vi "ILABs_CaseHandler.vi"(2 "error In":errorcluster, 3 "appReference":refnum<vi>, 4 "data":string, 5 "action":string) -> (0 "errorOut":string, 1 "response":string)   [LabVIEW 2009]
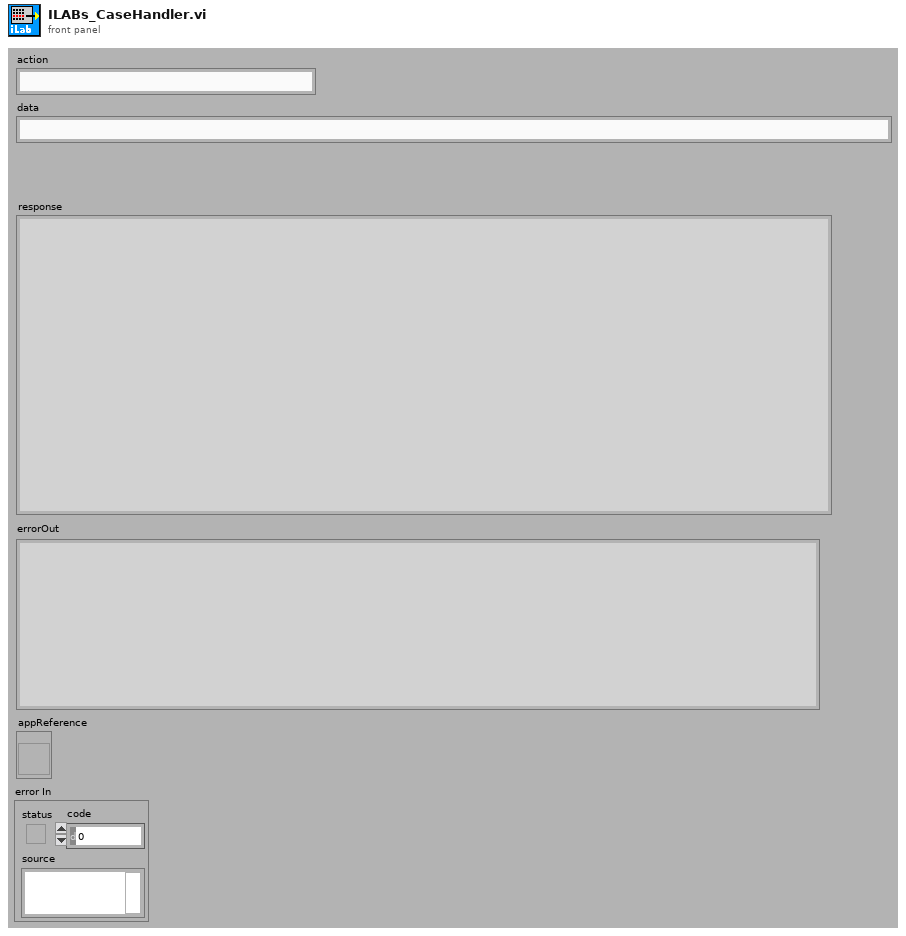
[diagram p1: front panel]
types:
  T1 = enum32{"Bad", "Idle", "Run top level", "Running"}
  T2 = typedef "LVRemotePanelConnectionsTypeDef.ctl" = cluster{"VI Name":string, "Remote":string, "UserName":string, "Port":i32, "Status":enum32{"Viewing", "Waiting For Control", "Controlling"}, "Create Time":timestamp, "Status Time":timestamp, "Control End Time":timestamp}[]
  T3 = cluster{"VI Name":string, "Remote":string, "UserName":string, "Port":i32, "Status":enum32{"Viewing", "Waiting For Control", "Controlling"}, "Create Time":timestamp, "Status Time":timestamp, "Control End Time":timestamp}
  T4 = cluster{"Name":string, "Path":path, "Type String":string, "Display Name":string, "Type":string}
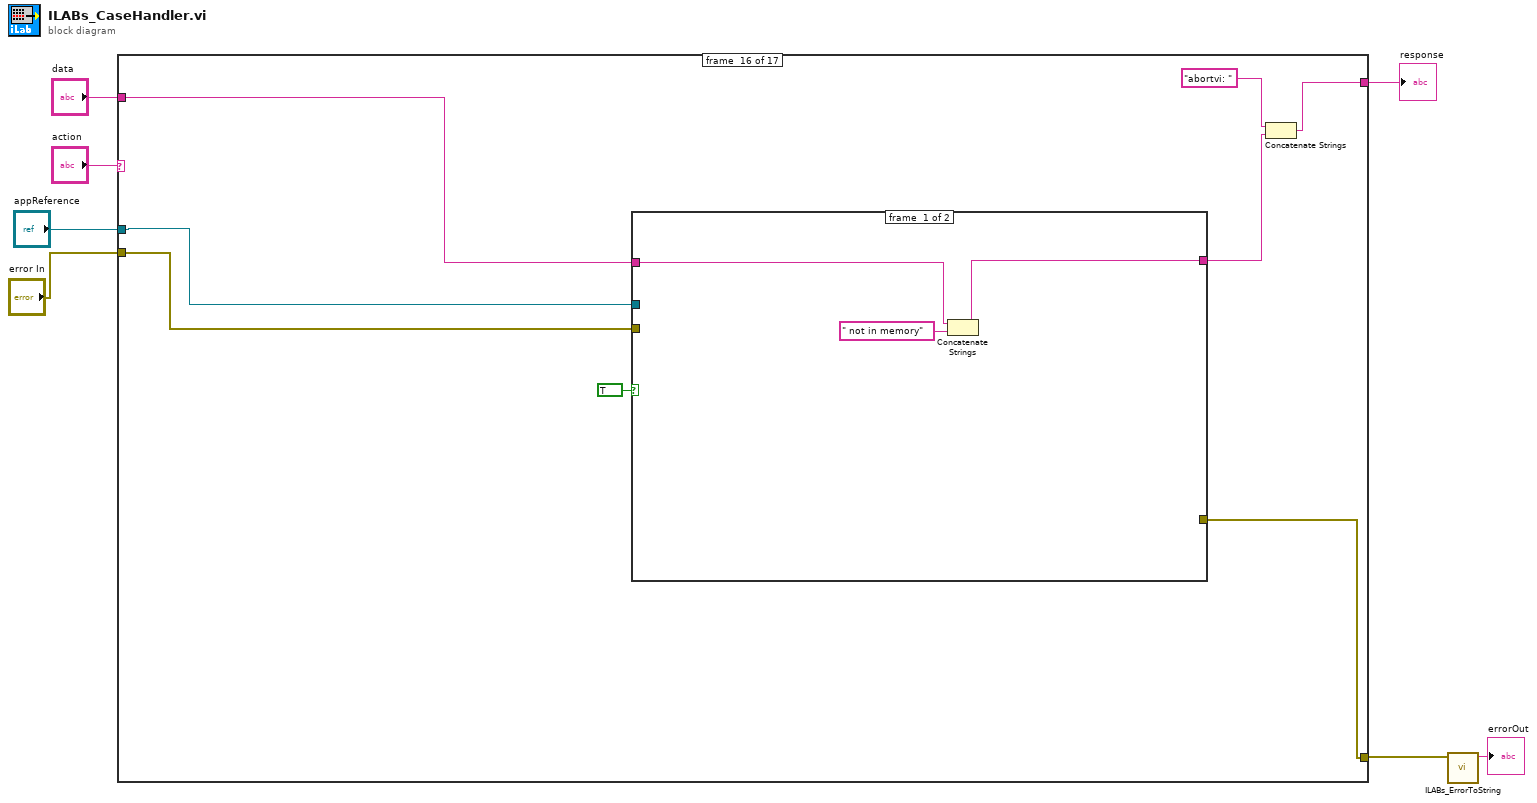
[diagram p0: block diagram]
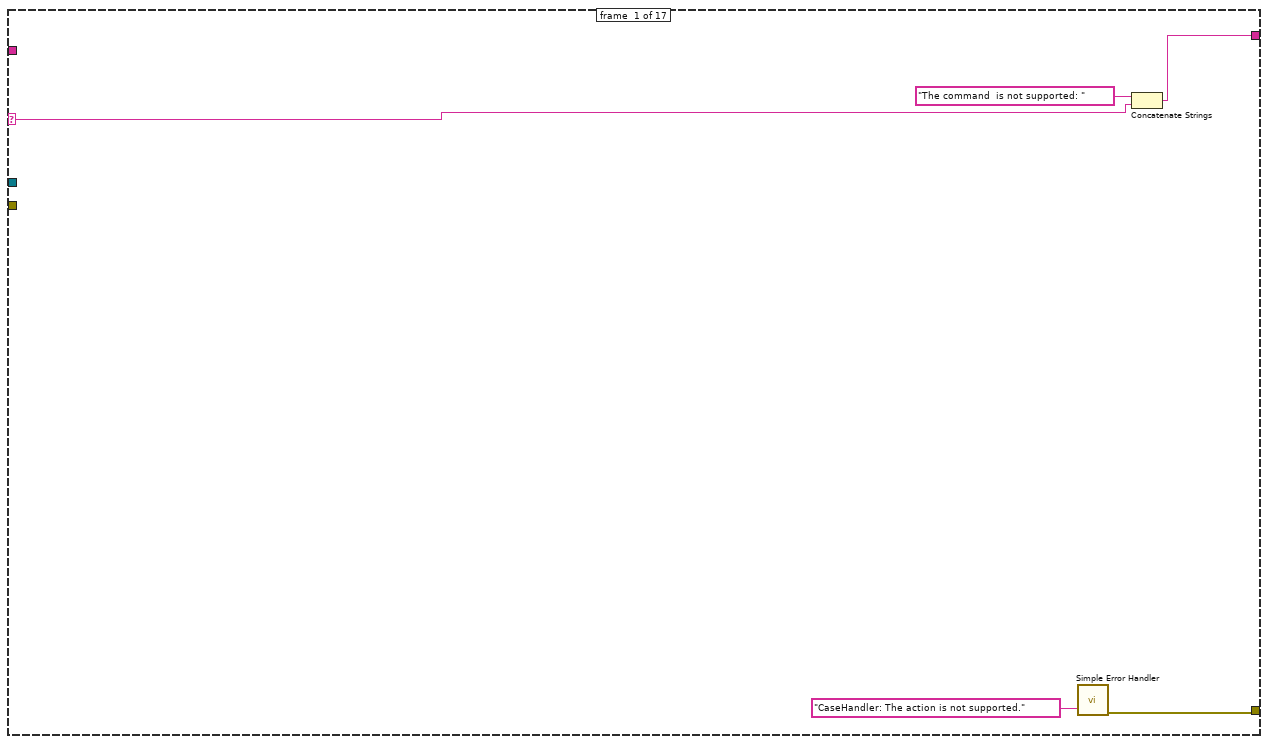
[diagram p2: hidden frame]
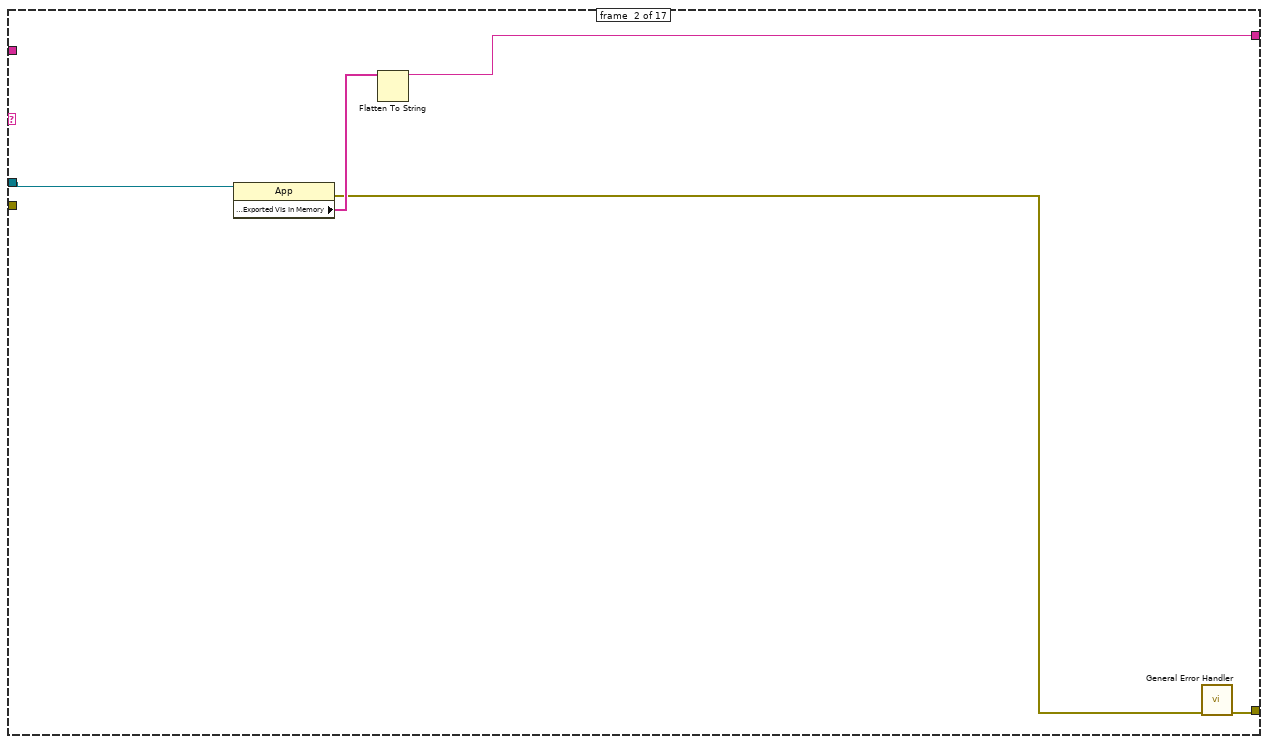
[diagram p3: hidden frame]
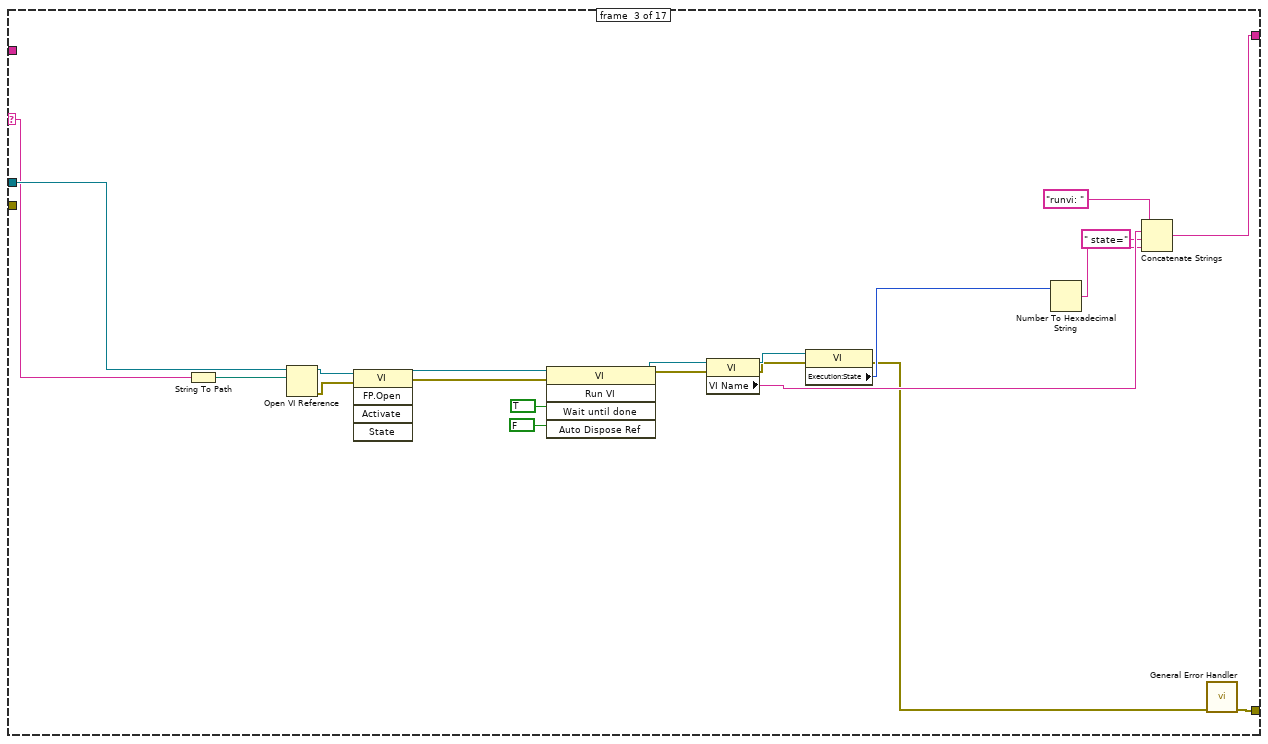
[diagram p4: hidden frame]
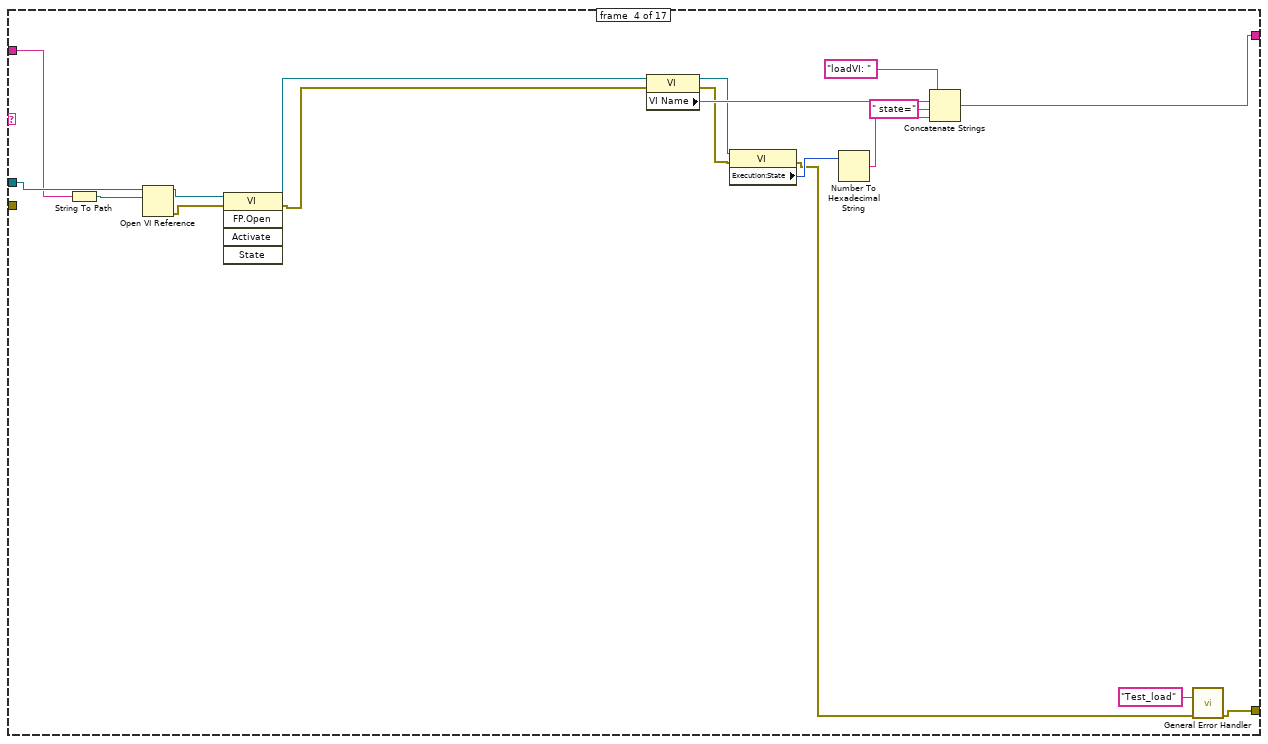
[diagram p5: hidden frame]
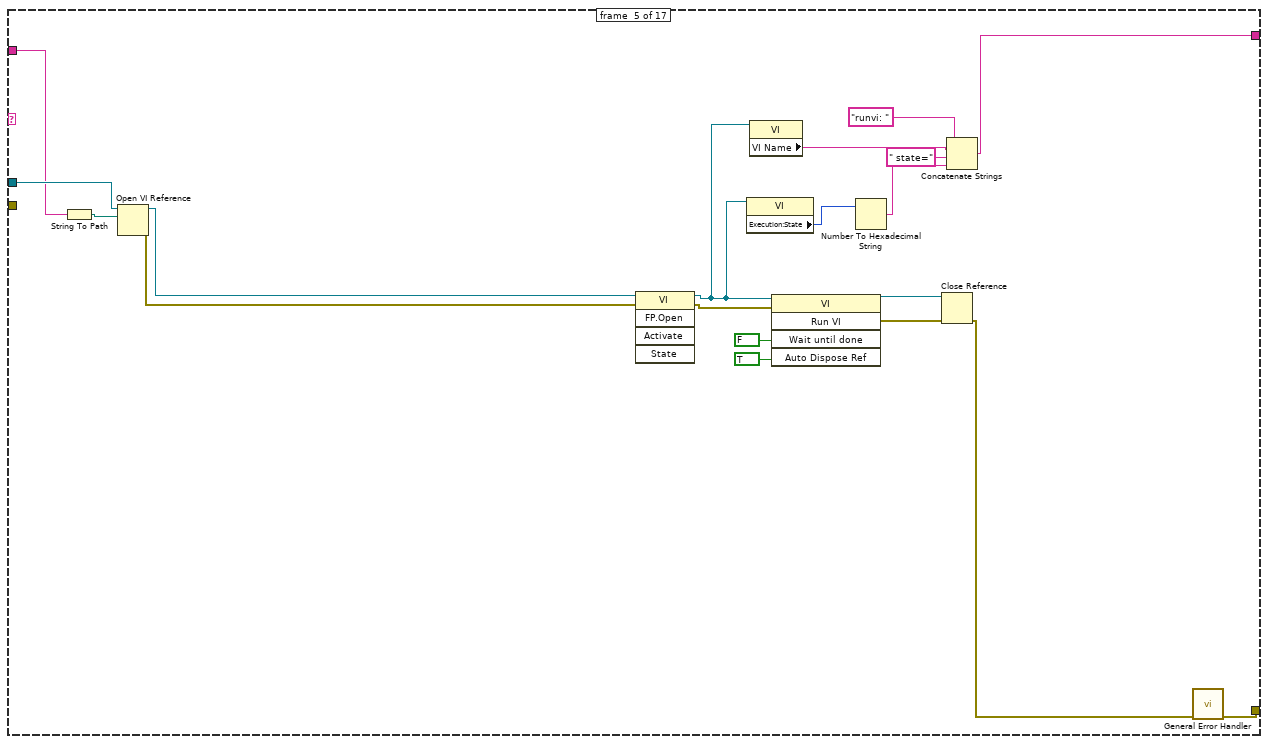
[diagram p6: hidden frame]
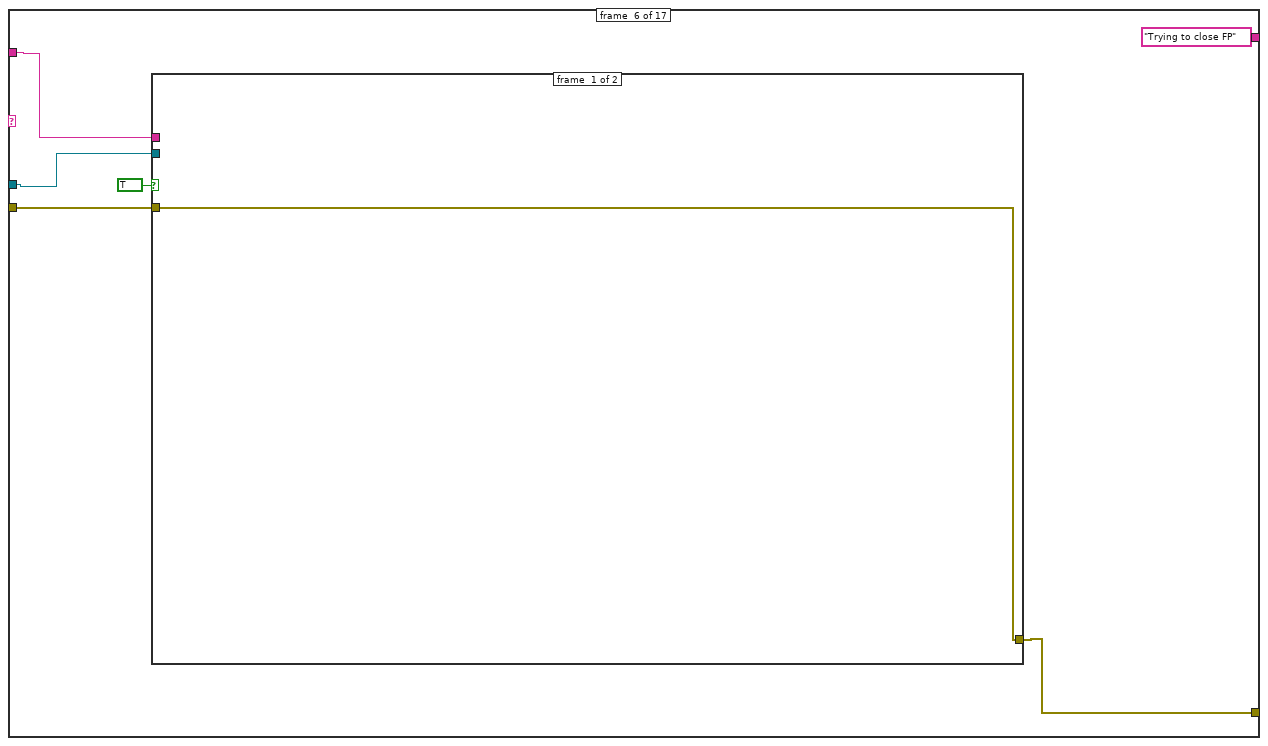
[diagram p7: hidden frame]
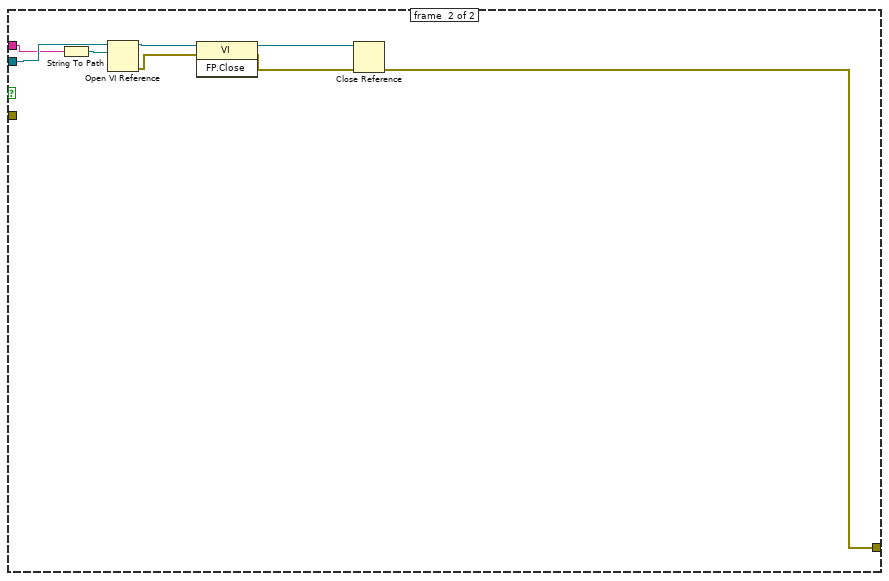
[diagram p8: hidden frame]
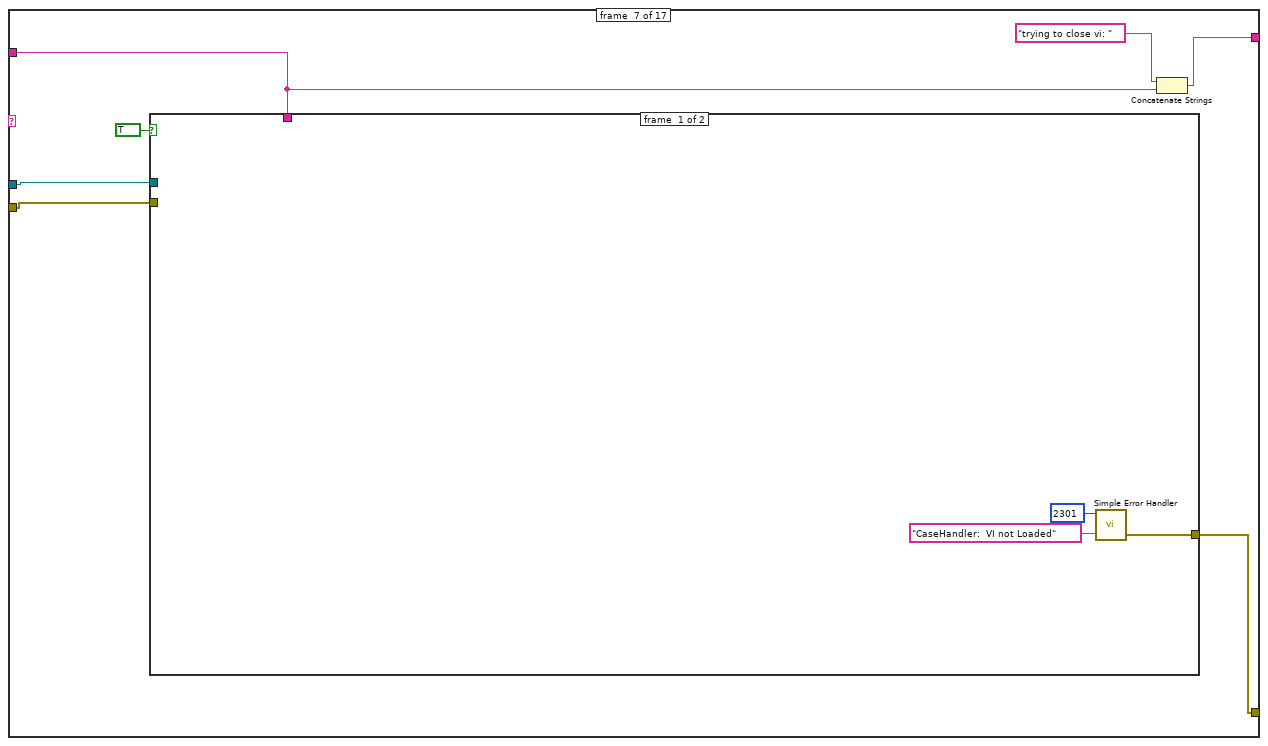
[diagram p9: hidden frame]
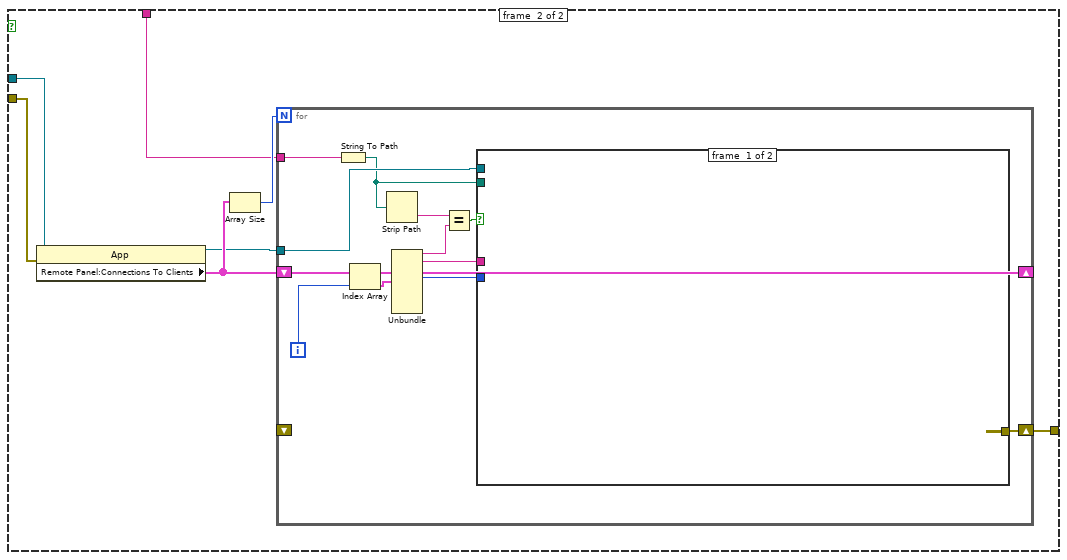
[diagram p10: hidden frame]
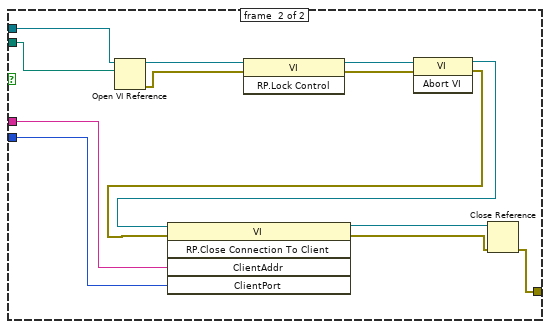
[diagram p11: hidden frame]
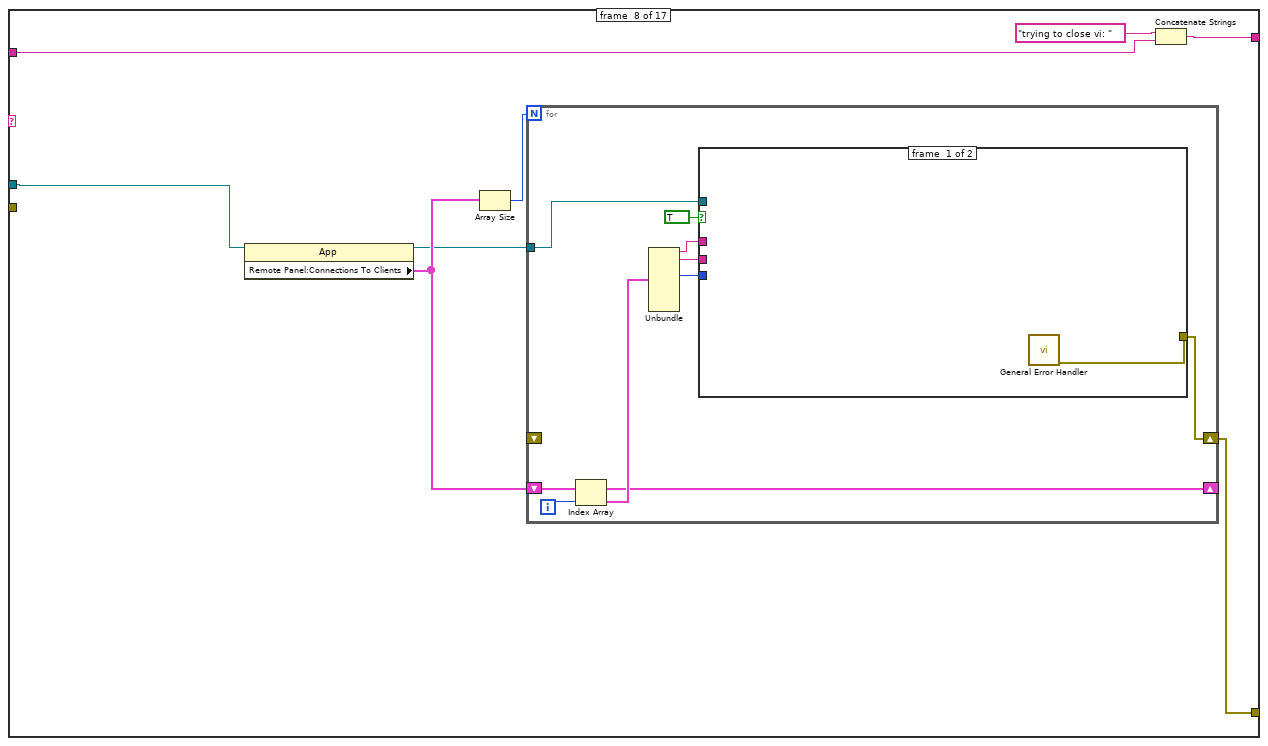
[diagram p12: hidden frame]
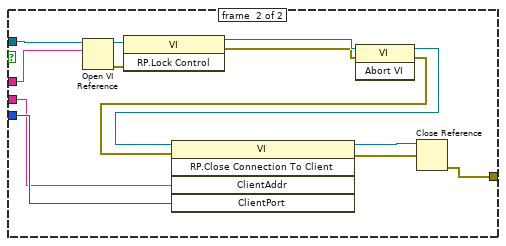
[diagram p13: hidden frame]
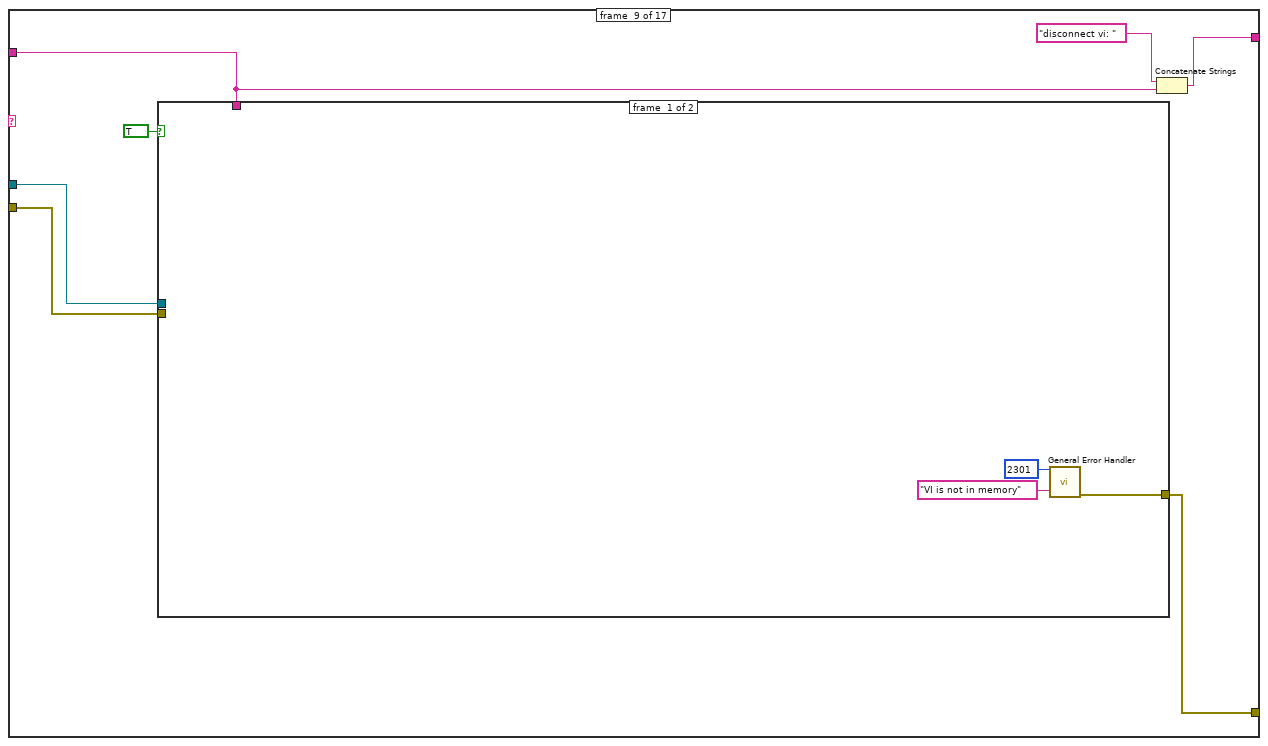
[diagram p14: hidden frame]
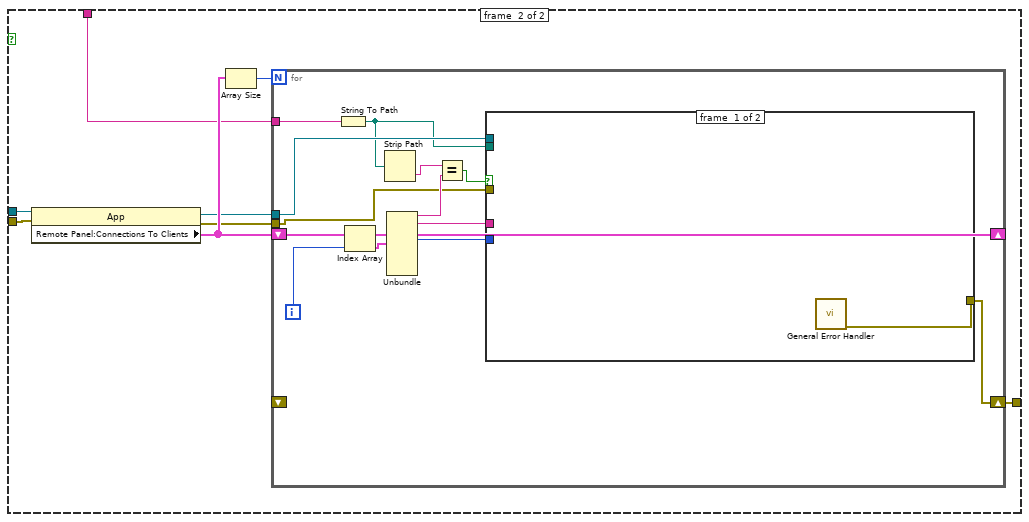
[diagram p15: hidden frame]
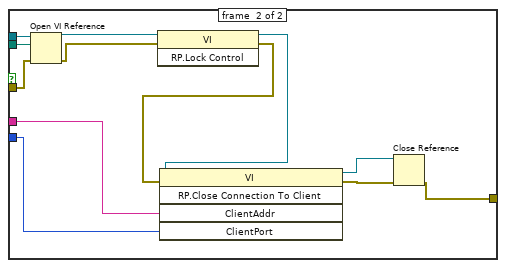
[diagram p16: hidden frame]
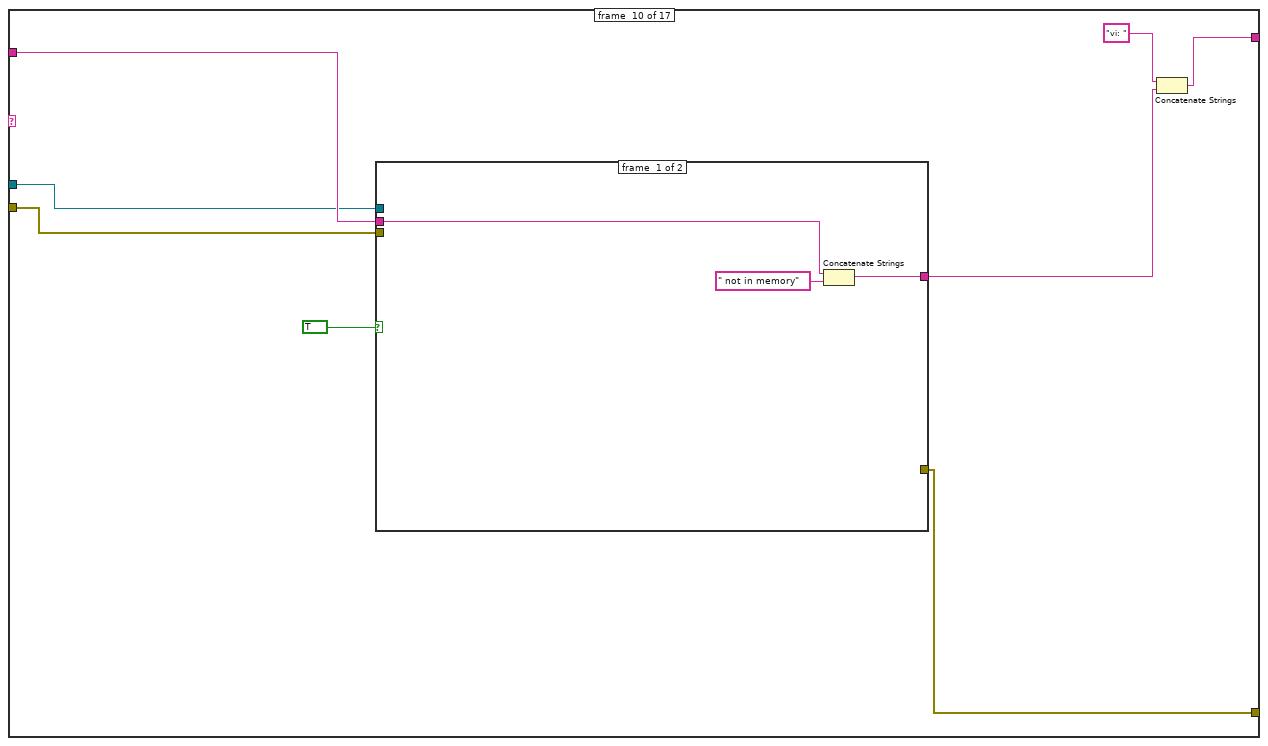
[diagram p17: hidden frame]
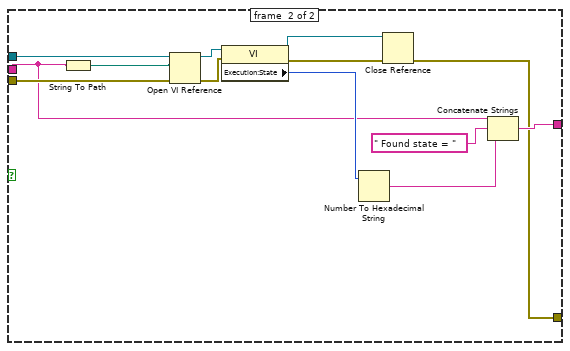
[diagram p18: hidden frame]
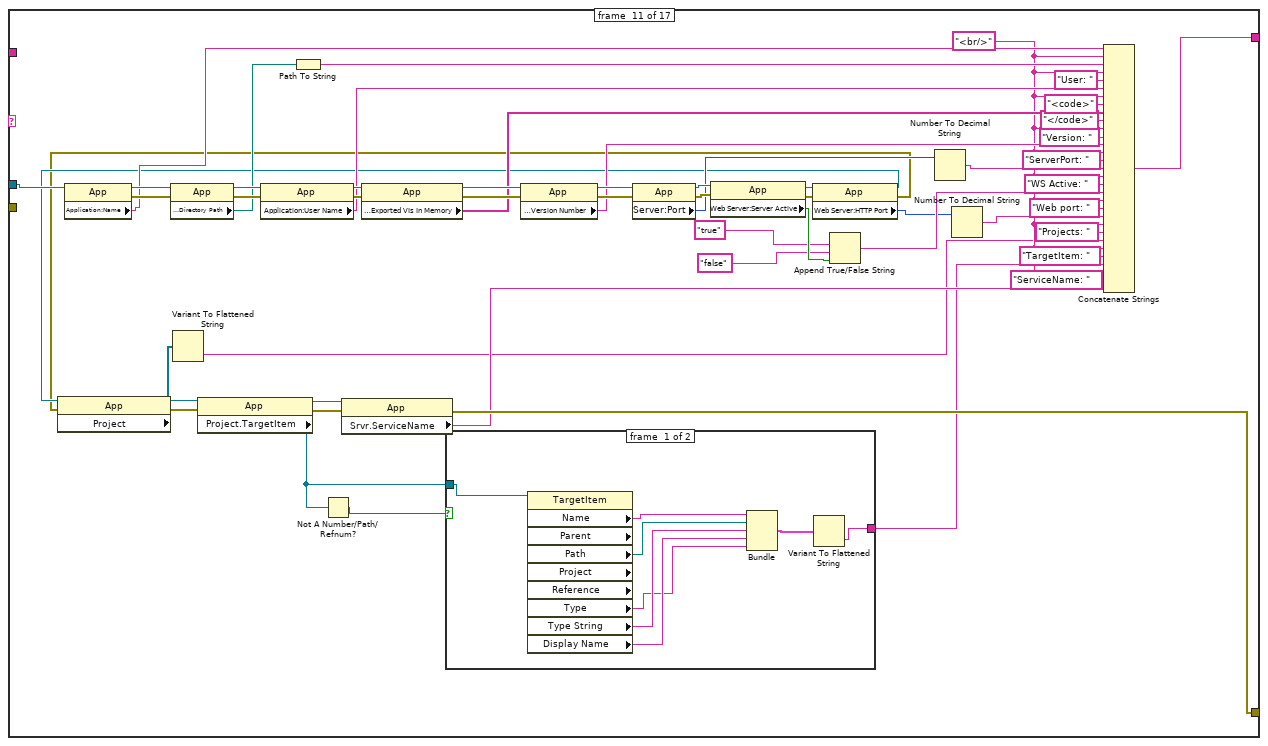
[diagram p19: hidden frame]
diagram:
  n1 = case shown="\"appstatus\"" "action" {
    selector: "action" -> [w11 _ w18 _ _ _ _ _ _ _ _ _ _ _ _ _ _]
    tunnel: "data" -> [_ _ _ w39 w57 w81 w94 w137 w167 w212 _ w295 w317 w327 w342 w370 w394]
    tunnel: [w10 w17 w30 w50 w66 "Trying to close FP" ("data") w96 w136 w169 w215 w249 w306 w326 w338 w346 w374 w394] -> w6
    tunnel: [w8 w14 w28 w49 w63 w79 w95 w135 w168 w211 w242 w297 w318 w329 w343 w371 _] -> w4
    tunnel: "appReference" -> [_ w13 w27 w48 w62 w80 w93 w134 w166 w210 w285 w294 w311 w330 w341 w369 _]
    tunnel: "error In" -> [_ _ _ _ _ w76 w92 _ w164 w209 _ w299 w312 _ w340 w368 _]
    frame #0 {
      (unwired) "The" ("message")
      n2 = call <vilib>:"Simple Error Handler.vi"("error source (\" \")"="CaseHandler: The action is not supported." ("error source (\" \")")) -> ("error out"=w8:errorcluster)  [unwired: 2 in, 6 out]
      n3 = Concatenate Strings("The command  is not supported: " ("string"), w11) -> (w10:string)
    }
    frame #1 {
      n4 = property class="App"(reference=w13) -> (error out=w15:errorcluster, "Application:Exported VIs In Memory"=w16:string[])  [unwired: 1 in, 1 out]
      n5 = Flatten To String(anything=w16) -> (data string=w17:string)  [unwired: 1 in, 4 out]
      n6 = call <vilib>:"General Error Handler.vi"("error in (no error)"=w15) -> ("error out"=w14:errorcluster)  [unwired: 1 in, 13 out]
    }
    frame #2 {
      n7 = String To Path(string=w18) -> (path=w19:path)
      n8 = Open VI Reference(application reference (local)=w27, vi path=w19) -> (vi reference=w37:refnum<vi>, error out=w36:errorcluster)  [unwired: 1 in, 3 out]
      n9 = invoke class="VI" method="FP.Open"(reference=w37, error in=w36) -> (reference out=w26:refnum<vi>, error out=w25:errorcluster)  [unwired: 3 in, 3 out]
      n10 = invoke class="VI" method="Run VI"(reference=w26, error in=w25, "Wait until done"=FALSE, "Auto Dispose Ref"=TRUE) -> (reference out=w24:refnum<vi>, error out=w23:errorcluster)  [unwired: 1 in, 3 out]
      n11 = property class="VI"(reference=w24, error in=w23) -> (reference out=w22:refnum<vi>, error out=w21:errorcluster, "VI Name"=w35:string)
      n12 = property class="VI"(reference=w22, error in=w21) -> (error out=w20:errorcluster, "Execution:State"=w33:T1)  [unwired: 1 out]
      n13 = Number To Hexadecimal String(2:w33) -> (0:w32:string)  [unwired: 1 out]
      n14 = Concatenate Strings("runvi: " ("string"), w35, " state=" ("string"), w32) -> (w30:string)
      n15 = call <vilib>:"General Error Handler.vi"("error in (no error)"=w20) -> ("error out"=w28:errorcluster)  [unwired: 1 in, 13 out]
    }
    frame #3 {
      n16 = String To Path(string=w39) -> (path=w40:path)
      n17 = Open VI Reference(application reference (local)=w48, vi path=w40) -> (vi reference=w44:refnum<vi>, error out=w43:errorcluster)  [unwired: 1 in, 3 out]
      n18 = invoke class="VI" method="FP.Open"(reference=w44, error in=w43) -> (reference out=w42:refnum<vi>, error out=w41:errorcluster)  [unwired: 3 in, 3 out]
      n19 = property class="VI"(reference=w42, error in=w41) -> (reference out=w46:refnum<vi>, error out=w47:errorcluster, "VI Name"=w55:string)
      n20 = property class="VI"(reference=w46, error in=w47) -> (error out=w45:errorcluster, "Execution:State"=w53:T1)  [unwired: 1 out]
      n21 = Number To Hexadecimal String(2:w53) -> (0:w52:string)  [unwired: 1 out]
      n22 = Concatenate Strings("loadVI: " ("string"), w55, " state=" ("string"), w52) -> (w50:string)
      n23 = call <vilib>:"General Error Handler.vi"("[error source] (\" \")"="Test_load" ("[error source] (\" \")"), "error in (no error)"=w45) -> ("error out"=w49:errorcluster)  [unwired: 1 in, 12 out]
    }
    frame #4 {
      w64 = TRUE items=["OFF", "ON", "OFF", "ON"] ("Auto Dispose Ref")
      n24 = String To Path(string=w57) -> (path=w58:path)
      n25 = Open VI Reference(application reference (local)=w62, vi path=w58) -> (vi reference=w74:refnum<vi>, error out=w72:errorcluster)  [unwired: 1 in, 3 out]
      n26 = invoke class="VI" method="FP.Open"(reference=w74, error in=w72) -> (reference out=w71:refnum<vi>, error out=w73:errorcluster)  [unwired: 3 in, 3 out]
      n27 = property class="VI"(reference=w71) -> ("Execution:State"=w68:T1)  [unwired: 1 in, 2 out]
      n28 = property class="VI"(reference=w71) -> ("VI Name"=w70:string)  [unwired: 1 in, 2 out]
      n29 = invoke class="VI" method="Run VI"(reference=w71, error in=w73, "Wait until done"=FALSE, "Auto Dispose Ref"=w64) -> (reference out=w59:refnum<vi>, error out=w60:errorcluster)  [unwired: 1 in, 3 out]
      n30 = Number To Hexadecimal String(2:w68) -> (0:w67:string)  [unwired: 1 out]
      n31 = Close Reference(reference=w59, error in (no error)=w60) -> (error out=w61:errorcluster)
      n32 = Concatenate Strings("runvi: " ("string"), w70, " state=" ("string"), w67) -> (w66:string)
      n33 = call <vilib>:"General Error Handler.vi"("error in (no error)"=w61) -> ("error out"=w63:errorcluster)  [unwired: 1 in, 13 out]
    }
    frame #5 {
      n34 = case shown="True" TRUE {
        tunnel: w81 -> [_ w83]
        tunnel: w80 -> [_ w90]
        tunnel: [w82 w85] -> w79
        tunnel: w76 -> [w82 _]
        frame #0 {
        }
        frame #1 {
          n35 = String To Path(string=w83) -> (path=w84:path)
          n36 = Open VI Reference(application reference (local)=w90, vi path=w84) -> (vi reference=w89:refnum<vi>, error out=w88:errorcluster)  [unwired: 1 in, 3 out]
          n37 = invoke class="VI" method="FP.Close"(reference=w89, error in=w88) -> (reference out=w87:refnum<vi>, error out=w86:errorcluster)  [unwired: 1 in, 1 out]
          n38 = Close Reference(reference=w87, error in (no error)=w86) -> (error out=w85:errorcluster)
        }
      }
    }
    frame #6 {
      n39 = case shown="True" TRUE {
        tunnel: [w100 w105] -> w95
        tunnel: w94 -> [_ w104]
        tunnel: w92 -> [_ w102]
        tunnel: w93 -> [_ w103]
        frame #0 {
          n40 = call <vilib>:"Simple Error Handler.vi"("error code (no error:0)"=2301, "error source (\" \")"="CaseHandler:  VI not Loaded" ("error source (\" \")")) -> ("error out"=w100:errorcluster)  [unwired: 2 in, 5 out]
        }
        frame #1 {
          n41 = property class="App"(reference=w103, error in=w102) -> (reference out=w101:refnum<vi>, "Remote Panel:Connections To Clients"=w106:T2)  [unwired: 1 out]
          n42 = Array Size(array=w106) -> (size(s)=w107:i32)
          n43 = for {
            N: w107 -> [_]
            shift-right: [w112] -> _
            shift-left: w106 -> [w112]
            tunnel: w104 -> [w109]
            shift-right: [w114] -> w105
            shift-left: _ -> [_]
            tunnel: w101 -> [w111]
            i -> [w119]
            n44 = String To Path(string=w109) -> (path=w108:path)
            n45 = Index Array(array=w112, index=w119) -> (element=w118:T3)
            n46 = Strip Path(path=w108) -> (name=w110:string)  [unwired: 1 out]
            n47 = Unbundle(w118) -> ("VI Name"=w113:string, "Remote"=w115:string, "Port"=w116:i32)  [unwired: 5 out]
            n48 = Equal?(x=w110, y=w113) -> (x = y?=w117:bool)
            n49 = case shown="True" w117 {
              tunnel: w116 -> [_ w132]
              tunnel: w115 -> [_ w131]
              tunnel: [_ w130] -> w114
              tunnel: w111 -> [_ w121]
              tunnel: w108 -> [_ w120]
              frame #0 {
              }
              frame #1 {
                n50 = Open VI Reference(application reference (local)=w121, vi path=w120) -> (vi reference=w129:refnum<vi>, error out=w128:errorcluster)  [unwired: 1 in, 3 out]
                n51 = invoke class="VI" method="RP.Lock Control"(reference=w129, error in=w128) -> (reference out=w127:refnum<vi>, error out=w126:errorcluster)  [unwired: 1 in, 1 out]
                n52 = invoke class="VI" method="Abort VI"(reference=w127, error in=w126) -> (reference out=w123:refnum<vi>, error out=w125:errorcluster)  [unwired: 1 in, 1 out]
                n53 = invoke class="VI" method="RP.Close Connection To Client"(reference=w123, error in=w125, "ClientAddr"=w131, "ClientPort"=w132) -> (reference out=w122:refnum<vi>, error out=w124:errorcluster)  [unwired: 1 in, 3 out]
                n54 = Close Reference(reference=w122, error in (no error)=w124) -> (error out=w130:errorcluster)
              }
            }
          }
        }
      }
      n55 = Concatenate Strings("trying to close vi: " ("data"), w94) -> (w96:string)
    }
    frame #7 {
      n56 = property class="App"(reference=w134) -> (reference out=w133:refnum<vi>, "Remote Panel:Connections To Clients"=w139:T2)  [unwired: 1 in, 1 out]
      n57 = Array Size(array=w139) -> (size(s)=w140:i32)
      n58 = for {
        N: w140 -> [_]
        shift-right: [w143] -> _
        shift-left: w139 -> [w143]
        shift-right: [w145] -> w135
        shift-left: _ -> [_]
        tunnel: w133 -> [w142]
        i -> [w149]
        n59 = Index Array(array=w143, index=w149) -> (element=w148:T3)
        n60 = Unbundle(w148) -> ("VI Name"=w144:string, "Remote"=w146:string, "Port"=w147:i32)  [unwired: 5 out]
        n61 = case shown="True" TRUE {
          tunnel: w147 -> [_ w163]
          tunnel: w146 -> [_ w162]
          tunnel: [w150 w161] -> w145
          tunnel: w144 -> [_ w160]
          tunnel: w142 -> [_ w151]
          frame #0 {
            n62 = call <vilib>:"General Error Handler.vi"() -> ("error out"=w150:errorcluster)  [unwired: 2 in, 13 out]
          }
          frame #1 {
            n63 = Open VI Reference(application reference (local)=w151, vi path=w160) -> (vi reference=w155:refnum<vi>, error out=w154:errorcluster)  [unwired: 1 in, 3 out]
            n64 = invoke class="VI" method="RP.Lock Control"(reference=w155, error in=w154) -> (reference out=w153:refnum<vi>, error out=w152:errorcluster)  [unwired: 1 in, 1 out]
            n65 = invoke class="VI" method="Abort VI"(reference=w153, error in=w152) -> (reference out=w156:refnum<vi>, error out=w157:errorcluster)  [unwired: 1 in, 1 out]
            n66 = invoke class="VI" method="RP.Close Connection To Client"(reference=w156, error in=w157, "ClientAddr"=w162, "ClientPort"=w163) -> (reference out=w159:refnum<vi>, error out=w158:errorcluster)  [unwired: 1 in, 3 out]
            n67 = Close Reference(reference=w159, error in (no error)=w158) -> (error out=w161:errorcluster)
          }
        }
      }
      n68 = Concatenate Strings("trying to close vi: " ("data"), w137) -> (w136:string)
    }
    frame #8 {
      n69 = case shown="True" TRUE {
        tunnel: [w173 w179] -> w168
        tunnel: w167 -> [_ w178]
        tunnel: w166 -> [_ w177]
        tunnel: w164 -> [_ w175]
        frame #0 {
          n70 = call <vilib>:"General Error Handler.vi"("[error code] (0)"=2301, "[error source] (\" \")"="VI is not in memory" ("[error source] (\" \")")) -> ("error out"=w173:errorcluster)  [unwired: 2 in, 11 out]
        }
        frame #1 {
          n71 = property class="App"(reference=w177, error in=w175) -> (reference out=w176:refnum<vi>, error out=w174:errorcluster, "Remote Panel:Connections To Clients"=w180:T2)
          n72 = Array Size(array=w180) -> (size(s)=w181:i32)
          n73 = for {
            N: w181 -> [_]
            shift-right: [w187] -> _
            shift-left: w180 -> [w187]
            tunnel: w178 -> [w183]
            shift-right: [w189] -> w179
            shift-left: _ -> [_]
            tunnel: w176 -> [w186]
            tunnel: w174 -> [w185]
            i -> [w194]
            n74 = String To Path(string=w183) -> (path=w182:path)
            n75 = Index Array(array=w187, index=w194) -> (element=w193:T3)
            n76 = Strip Path(path=w182) -> (name=w184:string)  [unwired: 1 out]
            n77 = Unbundle(w193) -> ("VI Name"=w188:string, "Remote"=w190:string, "Port"=w191:i32)  [unwired: 5 out]
            n78 = Equal?(x=w184, y=w188) -> (x = y?=w192:bool)
            n79 = case shown="True" w192 {
              tunnel: w191 -> [_ w207]
              tunnel: w190 -> [_ w206]
              tunnel: [w195 w198] -> w189
              tunnel: w186 -> [_ w201]
              tunnel: w185 -> [_ w197]
              tunnel: w182 -> [_ w196]
              frame #0 {
                n80 = call <vilib>:"General Error Handler.vi"() -> ("error out"=w195:errorcluster)  [unwired: 2 in, 13 out]
              }
              frame #1 {
                n81 = Open VI Reference(application reference (local)=w201, vi path=w196, error in (no error)=w197) -> (vi reference=w205:refnum<vi>, error out=w202:errorcluster)  [unwired: 3 out]
                n82 = invoke class="VI" method="RP.Lock Control"(reference=w205, error in=w202) -> (reference out=w204:refnum<vi>, error out=w203:errorcluster)  [unwired: 1 in, 1 out]
                n83 = invoke class="VI" method="RP.Close Connection To Client"(reference=w204, error in=w203, "ClientAddr"=w206, "ClientPort"=w207) -> (reference out=w199:refnum<vi>, error out=w200:errorcluster)  [unwired: 1 in, 3 out]
                n84 = Close Reference(reference=w199, error in (no error)=w200) -> (error out=w198:errorcluster)
              }
            }
          }
        }
      }
      n85 = Concatenate Strings("disconnect vi: " ("data"), w167) -> (w169:string)
    }
    frame #9 {
      n86 = case shown="True" TRUE {
        tunnel: w212 -> [w218 w220]
        tunnel: [_ w222] -> w211
        tunnel: [w217 w227] -> w213
        tunnel: w210 -> [_ w225]
        tunnel: w209 -> [_ w221]
        frame #0 {
          n87 = Concatenate Strings(w218, " not in memory" ("string")) -> (w217:string)
        }
        frame #1 {
          n88 = String To Path(string=w220) -> (path=w219:path)
          n89 = Open VI Reference(application reference (local)=w225, vi path=w219, error in (no error)=w221) -> (vi reference=w231:refnum<vi>, error out=w230:errorcluster)  [unwired: 3 out]
          n90 = property class="VI"(reference=w231, error in=w230) -> (reference out=w224:refnum<vi>, error out=w223:errorcluster, "Execution:State"=w229:T1)
          n91 = Number To Hexadecimal String(2:w229) -> (0:w228:string)  [unwired: 1 out]
          n92 = Close Reference(reference=w224, error in (no error)=w223) -> (error out=w222:errorcluster)
          n93 = Concatenate Strings(w220, " Found state = " ("string"), w228) -> (w227:string)
        }
      }
      n94 = Concatenate Strings("vi: " ("data"), w213) -> (w215:string)
    }
    frame #10 {
      w240 = "<br/>" ("string")
      n95 = property class="App"(reference=w285) -> (reference out=w284:refnum<vi>, error out=w279:errorcluster, "Application:Name"=w270:string)  [unwired: 1 in]
      n96 = property class="App"(reference=w284, error in=w279) -> (reference out=w283:refnum<vi>, error out=w278:errorcluster, "Application:Directory Path"=w268:path)
      n97 = property class="App"(reference=w283, error in=w278) -> (reference out=w282:refnum<vi>, error out=w277:errorcluster, "Application:User Name"=w266:string)
      n98 = Path To String(path=w268) -> (string=w269:string)
      n99 = property class="App"(reference=w282, error in=w277) -> (reference out=w281:refnum<vi>, error out=w276:errorcluster, "Application:Exported VIs In Memory"=w264:string[])
      n100 = property class="App"(reference=w281, error in=w276) -> (reference out=w280:refnum<vi>, error out=w275:errorcluster, "Application:Version Number"=w261:string)
      n101 = property class="App"(reference=w280, error in=w275) -> (reference out=w271:refnum<vi>, error out=w272:errorcluster, "Server:Port"=w258:u32)
      n102 = property class="App"(reference=w271, error in=w272) -> (reference out=w274:refnum<vi>, error out=w273:errorcluster, "Web Server:Server Active"=w256:bool)
      n103 = property class="App"(reference=w274, error in=w273) -> (reference out=w248:refnum<vi>, error out=w245:errorcluster, "Web Server:HTTP Port"=w251:u16)
      n104 = property class="App"(reference=w248, error in=w245) -> (reference out=w247:refnum<vi>, error out=w244:errorcluster, "Project"=w236:refnum<vi>[])
      n105 = Variant To Flattened String(Variant=w236) -> (data string=w235:string)  [unwired: 1 out]
      n106 = property class="App"(reference=w247, error in=w244) -> (reference out=w246:refnum<vi>, error out=w243:errorcluster, "Project.TargetItem"=w232:refnum<vi>)
      n107 = Not A Number/Path/Refnum?(number/path/refnum=w232) -> (NaN/Path/Refnum?=w233:bool)
      n108 = property class="App"(reference=w246, error in=w243) -> (error out=w242:errorcluster, "Srvr.ServiceName"=w237:string)  [unwired: 1 out]
      n109 = case shown="True" w233 {
        tunnel: [w287 _] -> w234
        tunnel: w232 -> [w286 _]
        frame #0 {
          n110 = property class="TargetItem" props=["Name", "Parent", "Path", "Project", "Reference", "Type", "Type String", "Display Name"](reference=w286) -> ("Name"=w293:string, "Path"=w292:path, "Type"=w289:string, "Type String"=w291:string, "Display Name"=w290:string)  [unwired: 1 in, 5 out]
          n111 = Bundle("Name"=w293, "Path"=w292, "Type String"=w291, "Display Name"=w290, "Type"=w289) -> (w288:T4)  [unwired: 1 out]
          n112 = Variant To Flattened String(Variant=w288) -> (data string=w287:string)  [unwired: 1 out]
        }
        frame #1 {
        }
      }
      n113 = Append True/False String(1:w256, 2:"false" ("false string"), 3:"true" ("true string")) -> (0:w255:string)  [unwired: 1 out]
      n114 = Number To Decimal String(number=w258) -> (decimal integer string=w259:string)  [unwired: 1 out]
      n115 = Number To Decimal String(number=w251) -> (decimal integer string=w250:string)  [unwired: 1 out]
      n116 = Concatenate Strings(w270, w240, w269, w240, "User: " ("string"), w266, w240, "<code>" ("string"), w264, "</code>" ("string"), w240, "Version: " ("string"), w261, w240, "ServerPort: " ("string"), w259, w240, "WS Active: " ("string"), w255, w240, "Web port: " ("string"), w250, w240, "Projects: " ("string"), w235, w240, "TargetItem: " ("string"), w234, w240, "ServiceName: " ("string"), w237) -> (w249:string)
    }
    frame #11 {
      n117 = String To Path(string=w295) -> (path=w296:path)
      n118 = Open VI Reference(application reference (local)=w294, vi path=w296, error in (no error)=w299) -> (vi reference=w304:refnum<vi>, error out=w303:errorcluster)  [unwired: 3 out]
      n119 = invoke class="VI" method="RP.Lock Control"(reference=w304, error in=w303) -> (reference out=w301:refnum<vi>, error out=w300:errorcluster)  [unwired: 1 in, 1 out]
      n120 = Close Reference(reference=w301, error in (no error)=w300) -> (error out=w297:errorcluster)
      n121 = Concatenate Strings(w295, ": lock Control requested " ("string")) -> (w298:string)
      n122 = Concatenate Strings("vi: " ("data"), w298) -> (w306:string)
    }
    frame #12 {
      n123 = property class="App"(reference=w311, error in=w312) -> (reference out=w310:refnum<vi>, error out=w307:errorcluster, "WebSrvr.Port"=w314:u16)
      n124 = String To Path(string=w317) -> (path=w316:path)
      n125 = Strip Path(path=w316) -> (name=w315:string)  [unwired: 1 out]
      n126 = invoke class="App" method="RP.Client Release Control"(reference=w310, error in=w307, "VIName"=w315, "ServerAddress"="thrush.mit.edu" ("Server Address"), "ServerPort"=w314) -> (reference out=w308:refnum<vi>, error out=w309:errorcluster)  [unwired: 1 in, 4 out]
      n127 = Open VI Reference(application reference (local)=w308, vi path=w316, error in (no error)=w309) -> (vi reference=w324:refnum<vi>, error out=w323:errorcluster)  [unwired: 3 out]
      n128 = invoke class="VI" method="RP.Lock Control"(reference=w324, error in=w323) -> (reference out=w321:refnum<vi>, error out=w320:errorcluster)  [unwired: 1 in, 1 out]
      n129 = Close Reference(reference=w321, error in (no error)=w320) -> (error out=w318:errorcluster)
      n130 = Concatenate Strings(w317, ": lock Control requested " ("string")) -> (w319:string)
      n131 = Concatenate Strings("vi: " ("data"), w319) -> (w326:string)
    }
    frame #13 {
      n132 = String To Path(string=w327) -> (path=w328:path)
      n133 = Open VI Reference(application reference (local)=w330, vi path=w328) -> (vi reference=w336:refnum<vi>, error out=w335:errorcluster)  [unwired: 1 in, 3 out]
      n134 = invoke class="VI" method="RP.Unlock Control"(reference=w336, error in=w335) -> (reference out=w333:refnum<vi>, error out=w332:errorcluster)  [unwired: 1 in, 1 out]
      n135 = Concatenate Strings(w327, ": unlock requested " ("string")) -> (w331:string)
      n136 = Close Reference(reference=w333, error in (no error)=w332) -> (error out=w329:errorcluster)
      n137 = Concatenate Strings("vi: " ("data"), w331) -> (w338:string)
    }
    frame #14 {
      n138 = case shown="True" TRUE {
        tunnel: w342 -> [w349 w357]
        tunnel: [_ w359] -> w343
        tunnel: [w348 w364] -> w344
        tunnel: w341 -> [_ w362]
        tunnel: w340 -> [_ w358]
        frame #0 {
          n139 = Concatenate Strings(w349, " not in memory" ("string")) -> (w348:string)
        }
        frame #1 {
          n140 = String To Path(string=w357) -> (path=w356:path)
          n141 = Open VI Reference(application reference (local)=w362, vi path=w356, error in (no error)=w358) -> (vi reference=w354:refnum<vi>, error out=w355:errorcluster)  [unwired: 1 in, 2 out]
          n142 = invoke class="VI" method="Ctrl Val.Set"(reference=w354, error in=w355, "Control Name"="stop", "Value"=TRUE) -> (reference out=w351:refnum<vi>, error out=w352:errorcluster)  [unwired: 1 in, 3 out]
          n143 = property class="VI"(reference=w351, error in=w352) -> (reference out=w361:refnum<vi>, error out=w360:errorcluster, "Execution:State"=w366:T1)
          n144 = Close Reference(reference=w361, error in (no error)=w360) -> (error out=w359:errorcluster)
          n145 = Number To Hexadecimal String(2:w366) -> (0:w365:string)  [unwired: 1 out]
          n146 = Concatenate Strings(w357, " Found state = " ("string"), w365) -> (w364:string)
        }
      }
      n147 = Concatenate Strings("stopvi: " ("data"), w344) -> (w346:string)
    }
    frame #15 {
      n148 = case shown="True" TRUE {
        tunnel: w370 -> [w377 w379]
        tunnel: [_ w383] -> w371
        tunnel: [w376 w390] -> w372
        tunnel: w369 -> [_ w386]
        tunnel: w368 -> [_ w380]
        frame #0 {
          n149 = Concatenate Strings(w377, " not in memory" ("string")) -> (w376:string)
        }
        frame #1 {
          n150 = String To Path(string=w379) -> (path=w378:path)
          n151 = Open VI Reference(application reference (local)=w386, vi path=w378, error in (no error)=w380) -> (vi reference=w382:refnum<vi>, error out=w381:errorcluster)  [unwired: 1 in, 2 out]
          n152 = invoke class="VI" method="Abort VI"(reference=w382, error in=w381) -> (reference out=w388:refnum<vi>, error out=w387:errorcluster)  [unwired: 1 in, 1 out]
          n153 = property class="VI"(reference=w388, error in=w387) -> (reference out=w385:refnum<vi>, error out=w384:errorcluster, "Execution:State"=w392:T1)
          n154 = Close Reference(reference=w385, error in (no error)=w384) -> (error out=w383:errorcluster)
          n155 = Number To Hexadecimal String(2:w392) -> (0:w391:string)  [unwired: 1 out]
          n156 = Concatenate Strings(w379, " Found state = " ("string"), w391) -> (w390:string)
        }
      }
      n157 = Concatenate Strings("abortvi: " ("data"), w372) -> (w374:string)
    }
    frame #16 {
      n158 = Quit LabVIEW(quit? (T)=TRUE) -> ()
    }
  }
  "response" <- w6
  n159 = call "ILABs_ErrorToString.vi"("errorIn"=w4) -> ("errorOut"=→"errorOut":string)  [unwired: 10 out]
